vi "Problem 15 - recursive.vi"(8 "error in (no error)":errorcluster) -> (0 "error out":errorcluster)   [LabVIEW 2021, in "Project Euler.lvlib"]
uses:
  Project Euler.lvlib
  LUT_element.ctl
  Utilities/Named Timers/Named Timers.lvlib
panel:
  out "no. of LUT elements":i32
  out "LUT out":T1[](array[typedef])
  out "recursivity counter out":u32
  in  "use LUT implementation?":enum16{"without_LUT", "with_LUT"}(ring)=enum."with_LUT"
  out "Answer = r(n,m)= number of routes":u64
  in  "n (number of nodes on a side)":u64=10
  out "Total execution time (ms)":u32
  # "Development\nControls or indicators that are useful for development or testing, but which are not outputs of the VI."
  # "Input\nInputs to the VI"
  # "Output\nOutputs of the VI"
  # "n = 14 took:\n145,041 ms with optimised backtracking algorithm\n241 ms with recursive implementation\n\nexecution time decreased by a factor of 600 (600 times improvement)"
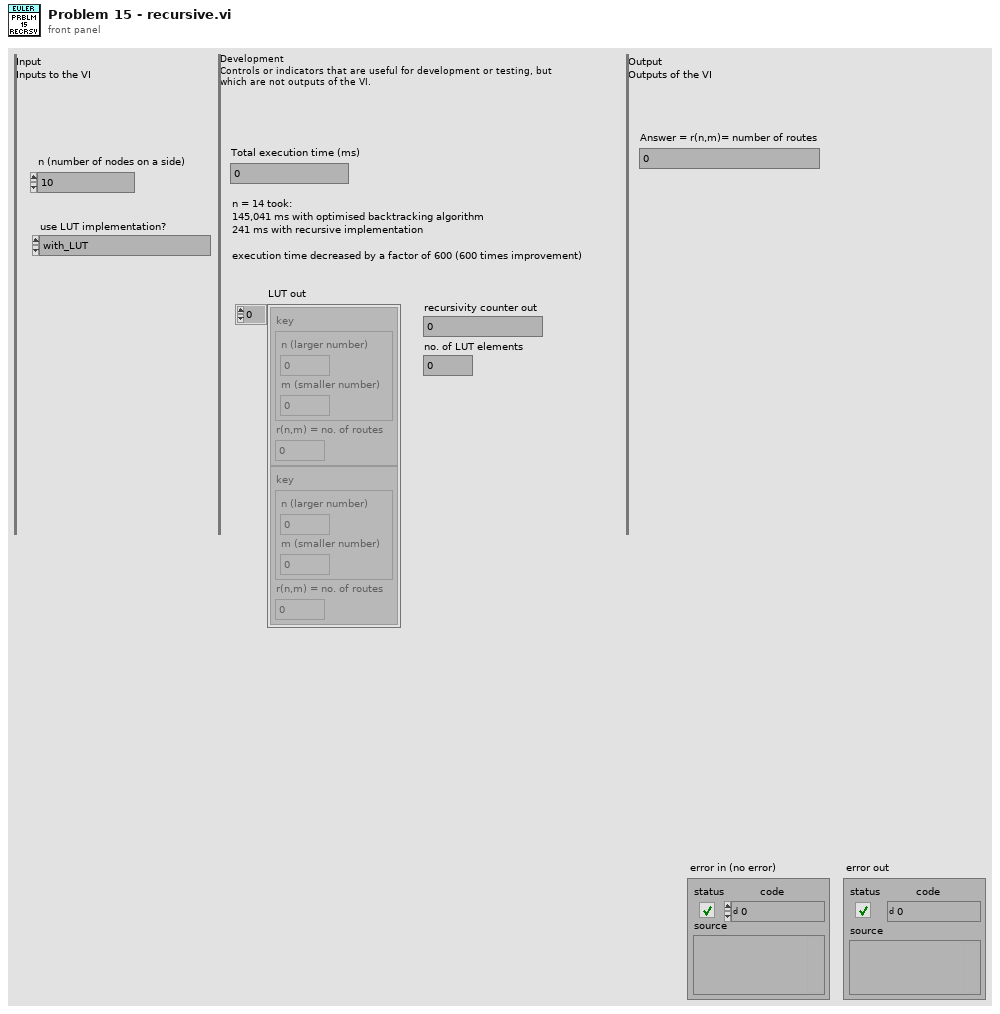
[diagram p1: front panel]
types:
  T1 = typedef "Project Euler.lvlib/LUT_element.ctl" = cluster{"key":cluster{"n (larger number)":u64, "m (smaller number)":u64}, "r(n,m) = no. of routes":u64}
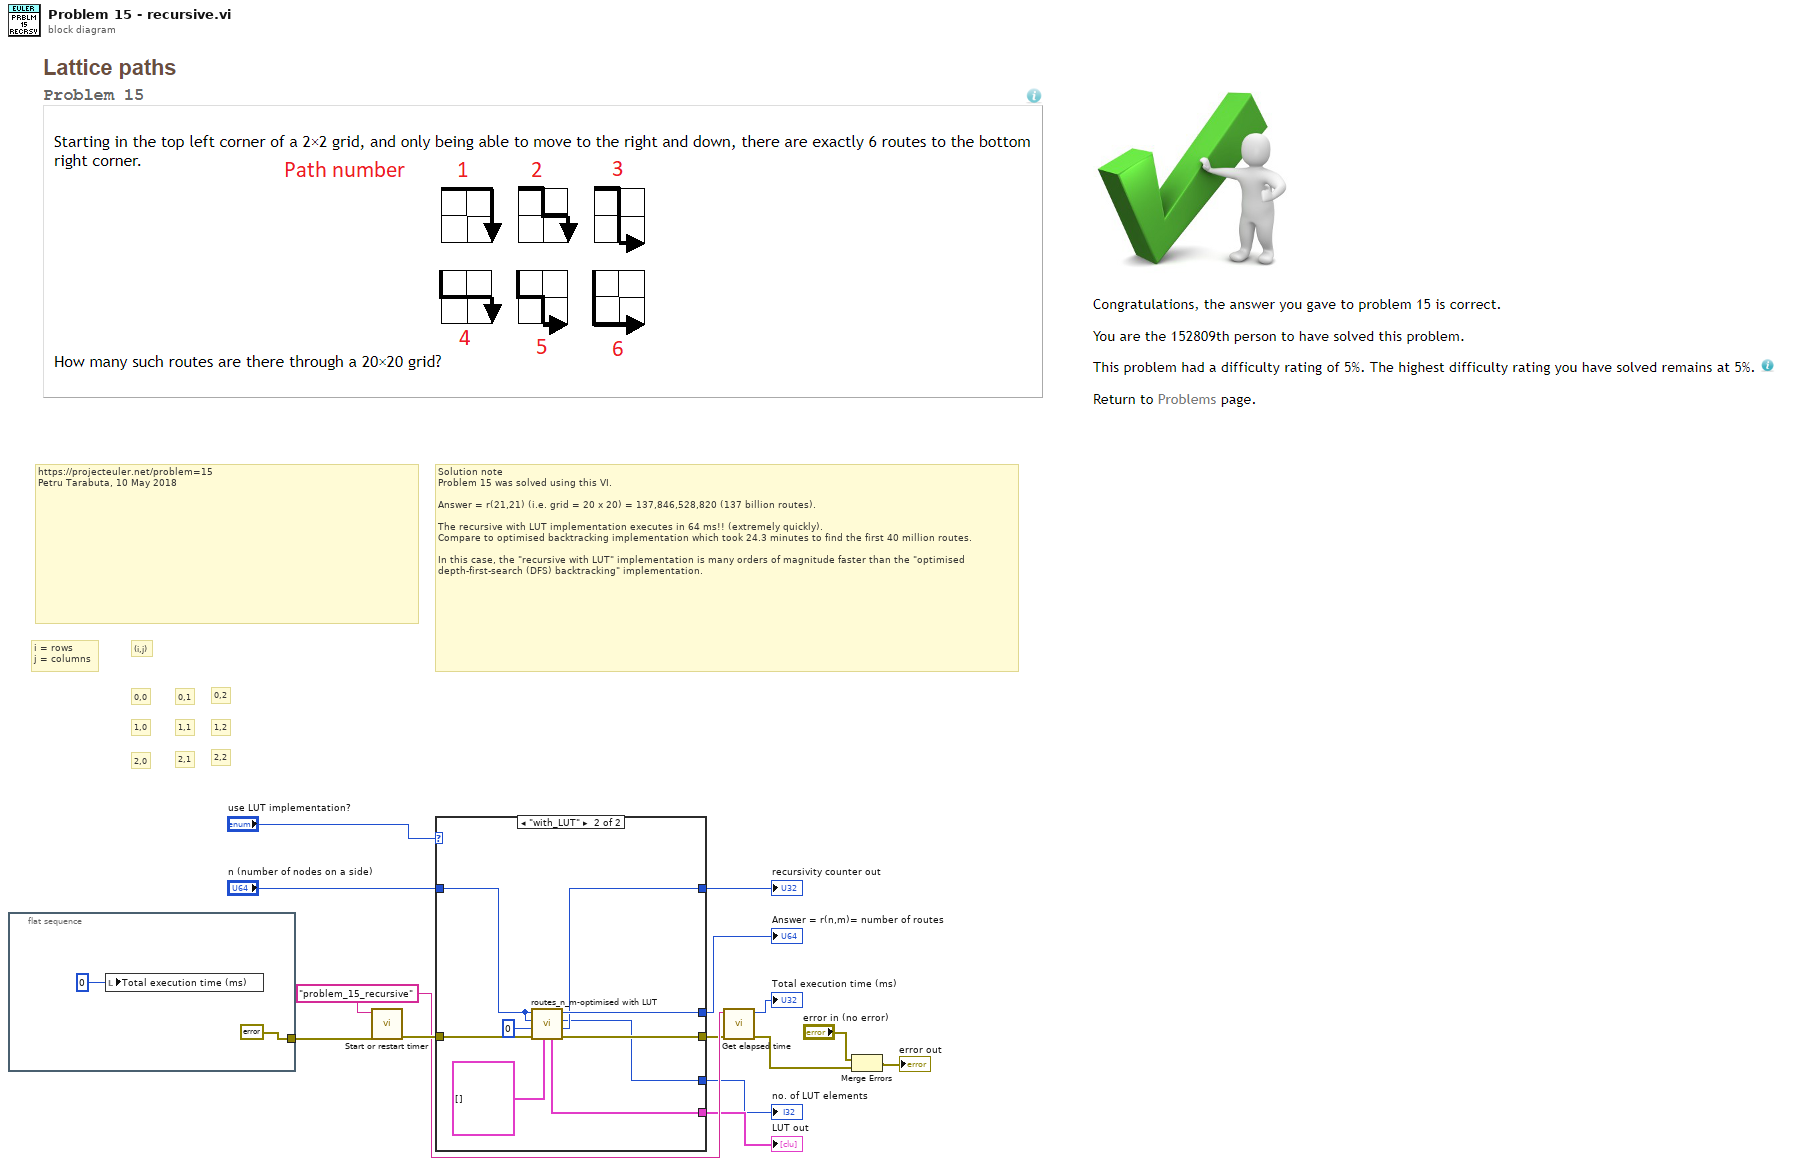
[diagram p0: block diagram]
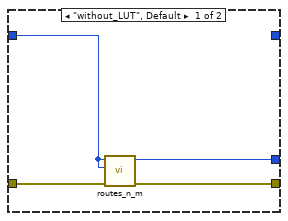
[diagram p2: hidden frame]
diagram:
  w7 = "problem_15_recursive" ("Timer name")
  # "Solution note\nProblem 15 was solved using this VI.\n\nAnswer = r(21,21) (i.e. grid = 20 x 20) = 137,846,528,820 (137 billion routes).\n\nThe recursive with LUT implementation executes in 64 ms!! (extremely quickly).\nCompare to optimised backtracking implementation which took 24.3 minutes to find the first 40 million routes.\n\nIn this case, the \"recursive with LUT\" implementation is many orders of magnitude faster than the \"optimised depth-first-search (DFS) backtracking\" implementation."
  # "2,2"
  # "2,1"
  # "1,2"
  # "1,1"
  # "0,2"
  # "0,1"
  # "2,0"
  # "(i,j)"
  # "i = rows\nj = columns"
  # "1,0"
  # "0,0"
  # "https://projecteuler.net/problem=15\nPetru Tarabuta, 10 May 2018"
  n1 = flat-sequence {
    tunnel: [w15] -> _
    tunnel: [w15] -> w13
    frame #0 {
      w15 = errorcluster {"status"=FALSE, "code"=0, "source"=""} ("error constant")
      n2 = local write "Total execution time (ms)"(u32 0 ("Total execution time (ms)")) -> ()
    }
  }
  n3 = call "Start or restart timer.vi"("error in (no error)"=w13, "Timer name"=w7) -> ("error out"=w8:errorcluster)  [unwired: 9 in]
  n4 = case shown="\"with_LUT\"" "use LUT implementation?" {
    tunnel: "n (number of nodes on a side)" -> [w20 w27]
    tunnel: w8 -> [w19 w29]
    tunnel: [w18 w28] -> w6
    tunnel: [w17 w26] -> w5
    tunnel: [_ w24] -> w3
    tunnel: [_ w22] -> w2
    tunnel: [_ w21] -> w1
    frame "without_LUT", Default {
      n5 = call "routes_n_m.vi"("error in (no error)"=w19, "m = number of nodes (horizontal)"=w20, "n = number of nodes (vertical)"=w20) -> ("error out"=w18:errorcluster, "r(n,m)= number of routes"=w17:u32)  [unwired: 7 in]
    }
    frame "with_LUT" {
      n6 = call "routes_n_m-optimised with LUT.vi"("LUT in"=T1[] [], "error in (no error)"=w29, "recursivity counter in"=u32 0, "m = number of nodes (horizontal)"=w27, "n = number of nodes (vertical)"=w27) -> ("error out"=w28:errorcluster, "recursivity counter out"=w24:u32, "no. of LUT elements"=w21:i32, "r(n,m)= number of routes"=w26:u64, "LUT out"=w22:T1[])  [unwired: 2 in]
    }
  }
  "Answer = r(n,m)= number of routes" <- w5
  "recursivity counter out" <- w3
  "LUT out" <- w2
  "no. of LUT elements" <- w1
  n7 = call "Get elapsed time.vi"("error in (no error)"=w6, "Timer name"=w7) -> ("error out"=w10:errorcluster, "Elapsed time (ms)"=→"Total execution time (ms)":u32)  [unwired: 6 in, 2 out]
  n8 = Merge Errors("error in (no error)", w10) -> (→"error out":errorcluster)
